vi "Plot2DArray.vi"() -> ()   [LabVIEW 2017]
panel:
  out "XY Graph":cluster{"Array":dbl[], "Array":dbl[]}(graph)
  in  "Array":dbl[][](array[numeric])
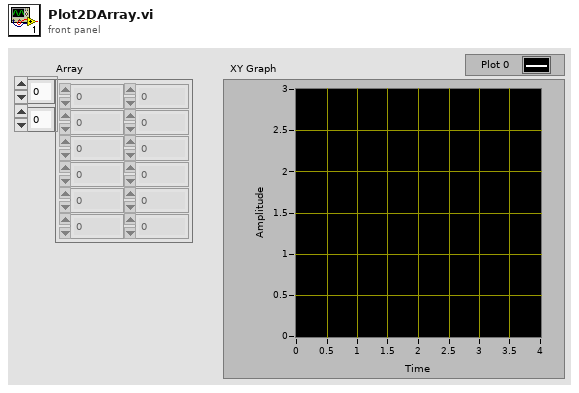
[diagram p1: front panel]
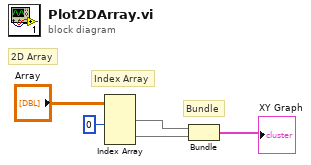
[diagram p0: block diagram]
diagram:
  # "2D Array"
  # "Index Array"
  # "Bundle"
  n1 = Index Array(array="Array", index (col) #1=0 ("disabled index (col)")) -> (element #1=w4:dbl[], element #2=w3:dbl[])  [unwired: 3 in]
  n2 = Bundle("Array"=w4, "Array"=w3) -> (→"XY Graph":cluster{"Array":dbl[], "Array":dbl[]})  [unwired: 1 in]
